vi "UpdateOwnerPath.vi"(11 "FileDependency in":map{path, T1}(c390)) -> (3 "FileDependency out":map{path, T1}(c390))   [LabVIEW 2020, in "DependencyViewer.lvlib"]
uses:
  DependencyViewer/DependencyViewer.lvlib
  FileDependencyType.ctl
  <vilib>/Utility/lvfile.llb/FT_FileTypes.ctl
  <vilib>/Utility/lvfile.llb/NI_FileType.lvlib
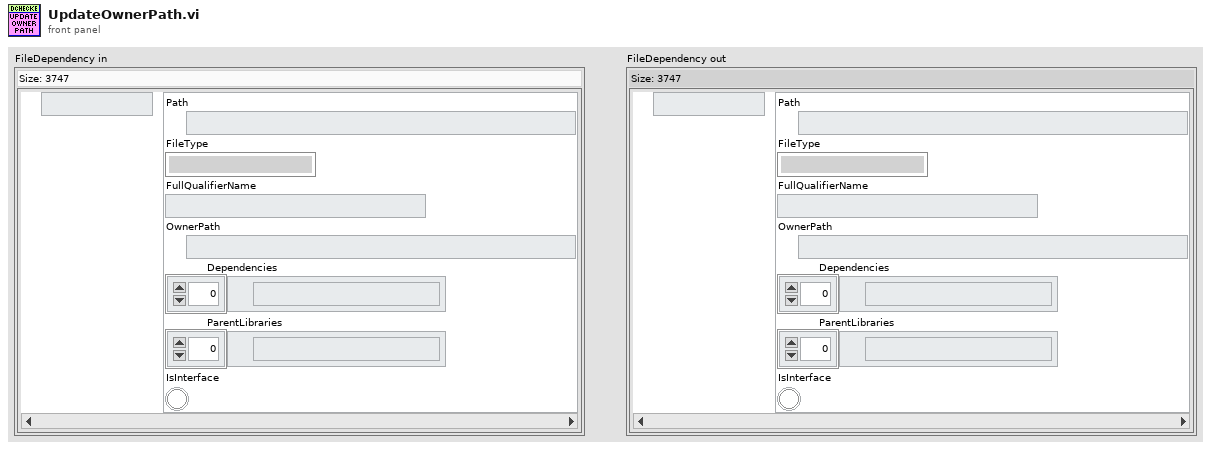
[diagram p1: front panel]
types:
  T1 = typedef "DependencyViewer.lvlib/FileDependencyType.ctl" = cluster{"Path":path, "FileType":T2, "FullQualifierName":string, "OwnerPath":path, "Dependencies":path[], "ParentLibraries":path[], "IsInterface":bool}
  T2 = typedef "NI_FileType.lvlib/FT_FileTypes.ctl" = enum32{"Invalid file/path", "Unknown type", "Instrument", "Control", "Polymorphic VI", "Project", "Library", "LVClass", "XControl", "XNode", "CIN", "Run-time menu", "Palette menu", "LLB", "Shortcut", "Directory", "Class Private Data Control", "Statechart", "MathScript .m file", "Ladder Diagram", "LVLibp"}
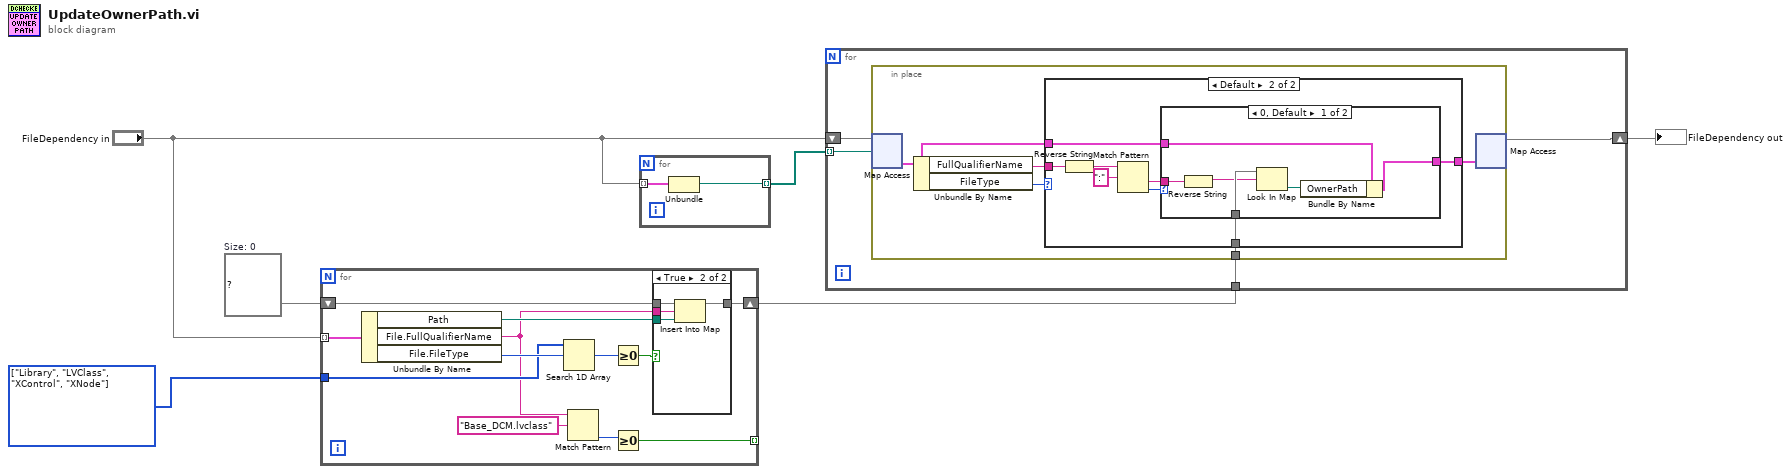
[diagram p0: block diagram]
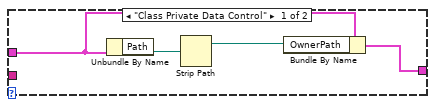
[diagram p2: hidden frame]
diagram:
  w5 = map{string, path} {}  # Size: 0
  w6 = T2[] [enum."Library", enum."LVClass", enum."XControl", enum."XNode"] items=["Invalid file/path", "Unknown type", "Instrument", "Control", "Polymorphic VI", "Project", "Library", "LVClass", "XControl", "XNode", "CIN", "Run-time menu", "Palette menu", "LLB", "Shortcut", "Directory", "Class Private Data Control", "Statechart", "MathScript .m file", "Ladder Diagram", "LVLibp"] ("y")
  n1 = for {
    tunnel: "FileDependency in" -> [w18] mode=indexing
    tunnel: w6 -> [w16]
    shift-right: [w13] -> w2
    shift-left: w5 -> [w14]
    tunnel: [w7] -> _ mode=indexing
    n2 = Unbundle By Name(w18) -> ("Path"=w12:path, "File.FullQualifierName"=w10:string, "File.FileType"=w17:T2)
    n3 = Search 1D Array(1D array=w16, element=w17) -> (index of element=w15:i32)  [unwired: 1 in]
    n4 = Match Pattern(string=w10, regular expression="Base_DCM.lvclass") -> (offset past match=w8:i32)  [unwired: 1 in, 3 out]
    n5 = Greater Or Equal To 0?(x=w15) -> (x >= 0?=w11:bool)
    n6 = Greater Or Equal To 0?(x=w8) -> (x >= 0?=w7:bool)
    n7 = case shown="True" w11 {
      tunnel: w14 -> [w19 w23]
      tunnel: [w19 w22] -> w13
      tunnel: w10 -> [_ w21]
      tunnel: w12 -> [_ w20]
      frame False {
      }
      frame True {
        n8 = Insert Into Map(map in=w23, key=w21, value=w20) -> (map out=w22:map{string, path})  [unwired: 2 out]
      }
    }
  }
  n9 = for {
    tunnel: "FileDependency in" -> [w25] mode=indexing
    tunnel: [w24] -> w3 mode=indexing
    n10 = Unbundle(w25) -> ("Path"=w24:path)  [unwired: 1 out]
  }
  n11 = for {
    shift-right: [w26] -> w1
    shift-left: "FileDependency in" -> [w29]
    tunnel: w3 -> [w28] mode=indexing
    tunnel: w2 -> [w27]
    n12 = in-place {
      in-place-border: w27 -> [w31]
      n13 = in-place-map #1(w29, w28) -> (w32:T1)  [unwired: 1 in, 1 out]
      n14 = Unbundle By Name(w32) -> ("FullQualifierName"=w34:string, "FileType"=w30:T2)
      n15 = case shown="Default" w30 {
        tunnel: w34 -> [_ w46]
        tunnel: [w35 w42] -> w33
        tunnel: w32 -> [w38 w41]
        tunnel: w31 -> [_ w39]
        frame "Class Private Data Control" {
          n16 = Unbundle By Name(w38) -> ("Path"=w37:path)
          n17 = Strip Path(path=w37) -> (stripped path=w36:path)  [unwired: 1 out]
          n18 = Bundle By Name(cluster=w38, "OwnerPath"=w36) -> (w35:T1)
        }
        frame Default {
          n19 = Reverse String(1:w46) -> (0:w45:string)
          n20 = Match Pattern(string=w45, regular expression=":") -> (after substring=w40:string, offset past match=w43:i32)  [unwired: 1 in, 2 out]
          n21 = case shown="0, Default" w43 {
            tunnel: [w47 w53] -> w42
            tunnel: w41 -> [w49 w53]
            tunnel: w40 -> [w52 _]
            tunnel: w39 -> [w51 _]
            frame 0, Default {
              n22 = Reverse String(1:w52) -> (0:w50:string)
              n23 = Look In Map(map=w51, key=w50) -> (value=w48:path)  [unwired: 1 in, 1 out]
              n24 = Bundle By Name(cluster=w49, "OwnerPath"=w48) -> (w47:T1)
            }
            frame -1 {
            }
          }
        }
      }
      n25 = in-place-map #1(w33) -> (w26:map{path, T1})  [unwired: 1 in, 2 out]
    }
  }
  "FileDependency out" <- w1
